vi "read_mote.vi"() -> (0 "DataSocket error":errorcluster, 1 "SF error":errorcluster, 3 "Timestamp":string)   [LabVIEW 2011]
panel:
  out "Location":string
  out "# Sent Data":u64
  out "Data comming from mote":string
  out "Deque error":errorcluster
  # "DO NOT USE id 0 for a mote !"
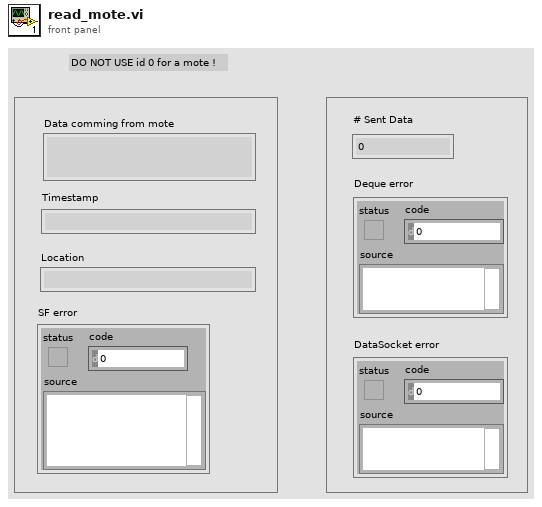
[diagram p1: front panel]
types:
  T1 = enum16{"Read", "Write", "ReadWrite", "BufferedRead", "BufferedReadWrite"}
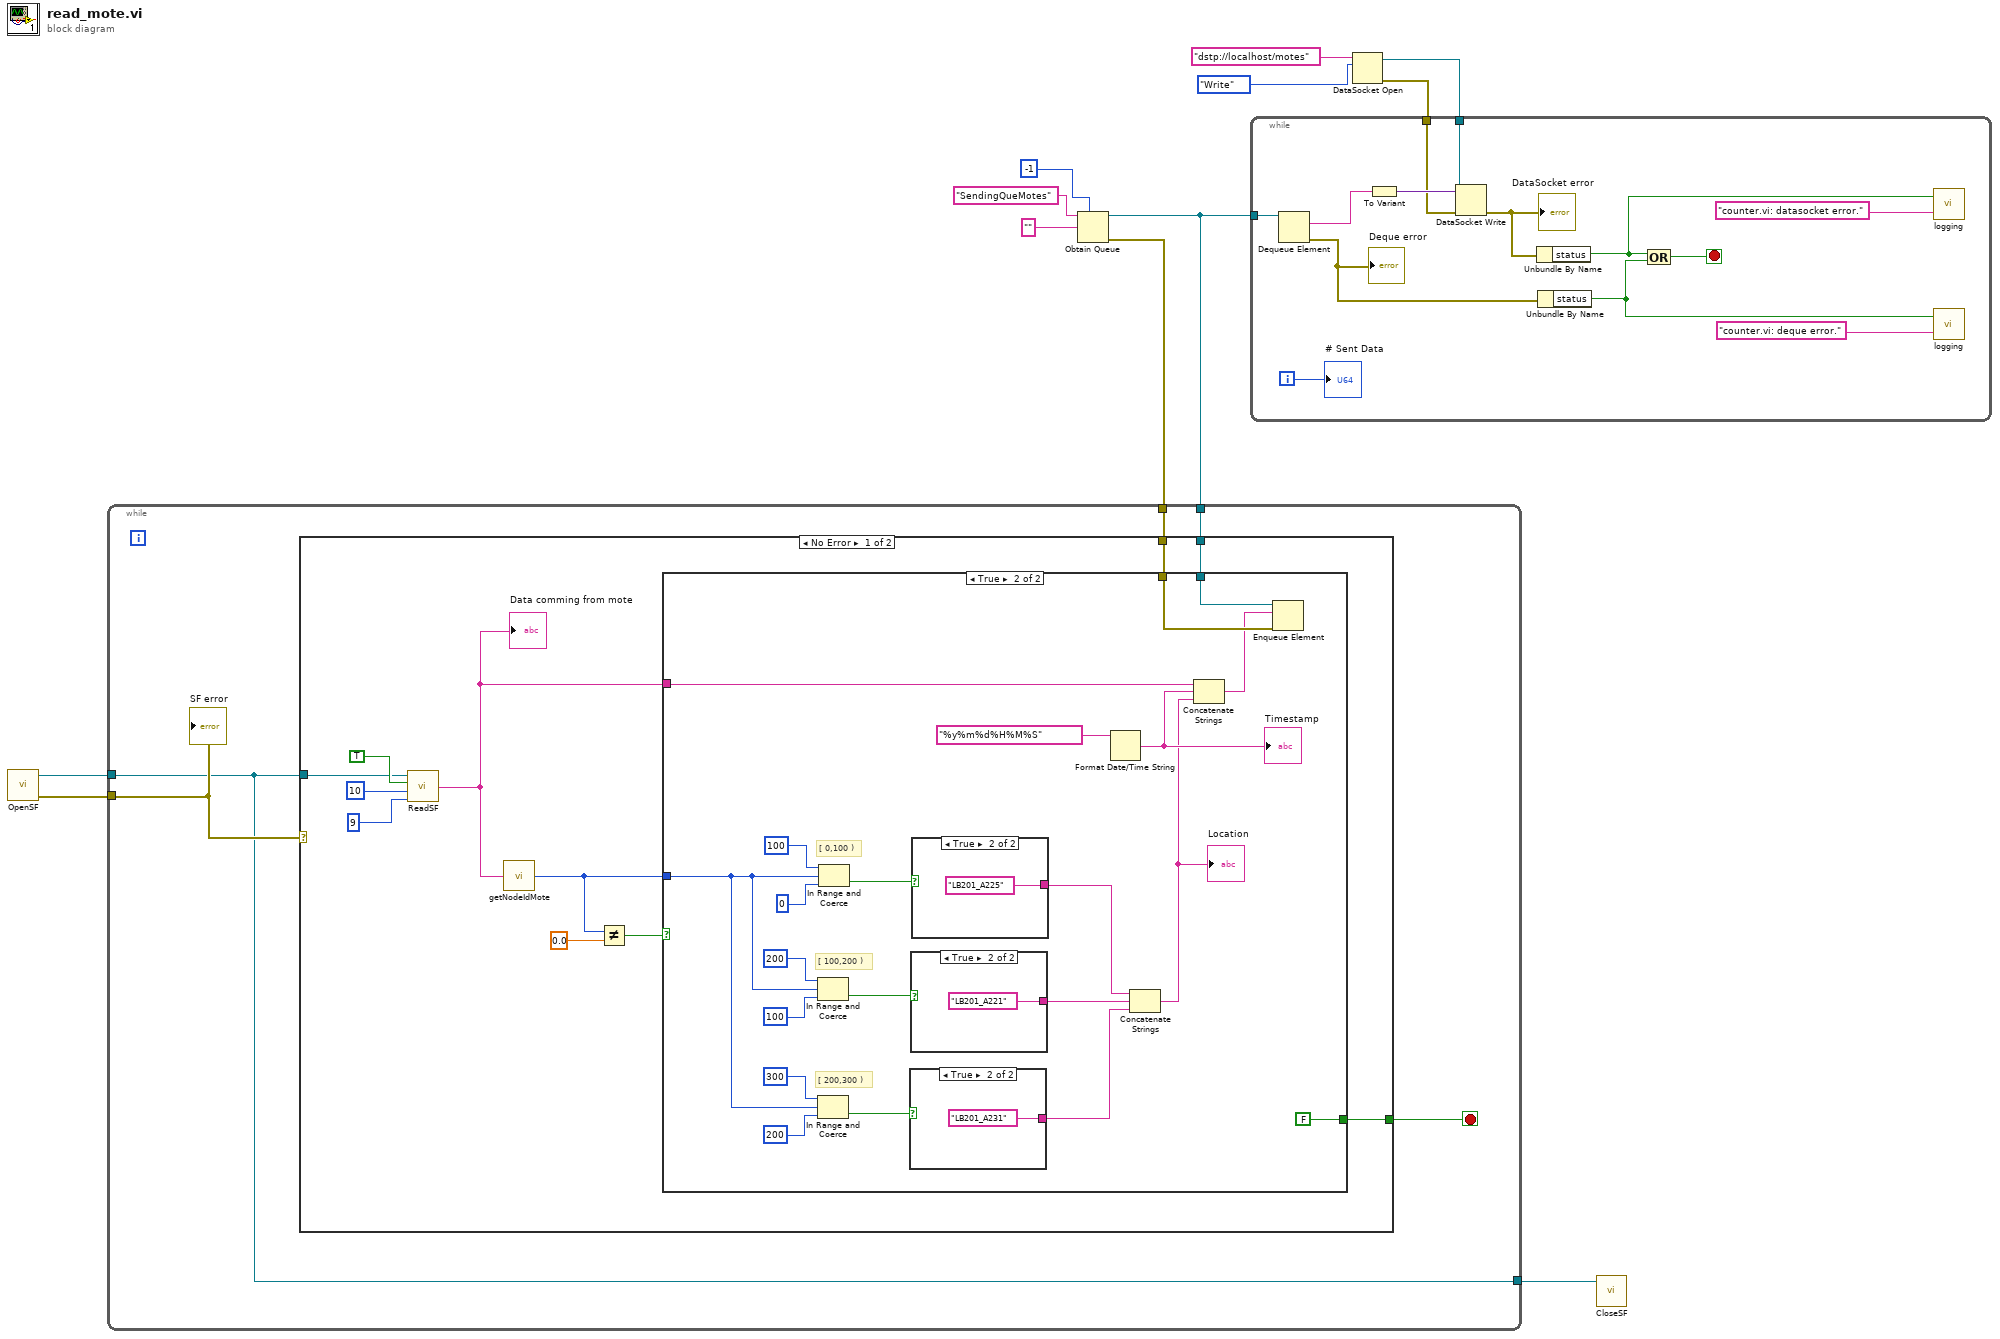
[diagram p0: block diagram]
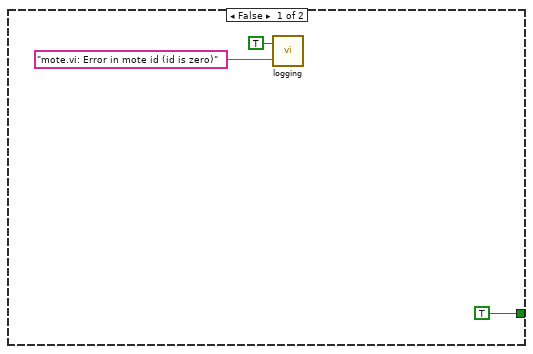
[diagram p2: hidden frame]
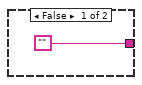
[diagram p3: hidden frame]
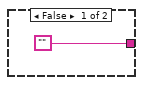
[diagram p4: hidden frame]
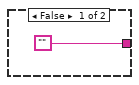
[diagram p5: hidden frame]
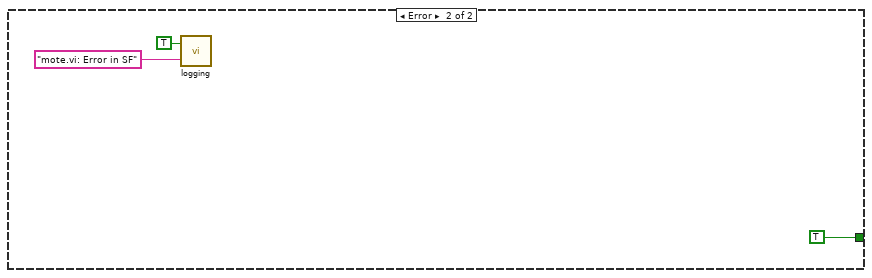
[diagram p6: hidden frame]
diagram:
  n1 = call "OpenSF.vi"() -> ("error out"=w3:errorcluster, "connection ID"=w2:refnum<k5>)  [unwired: 1 out]
  n2 = Obtain Queue(max queue size (-1, unlimited)=-1, name (unnamed)="SendingQueMotes", element data type="") -> (queue out=w5:refnum<queue>, error out=w6:errorcluster)  [unwired: 2 in, 1 out]
  n3 = while {
    tunnel: w2 -> [w14]
    tunnel: w3 -> [w15]
    tunnel: w6 -> [w17]
    tunnel: w5 -> [w16]
    tunnel: [w14] -> w1
    stop <- w13 stop-if-true
    n4 = case shown="No Error" w15 {
      tunnel: w14 -> [w25 _]
      tunnel: w17 -> [w24 _]
      tunnel: w16 -> [w23 _]
      tunnel: [w18 TRUE] -> w13
      frame No Error {
        n5 = call "ReadSF.vi"("connection ID in"=w25, "enabled"=TRUE, "bytes to read"=10 ("f"), "header size"=9 ("bytes to read")) -> ("string"=w22:string)  [unwired: 2 in, 2 out]
        "Data comming from mote" <- w22
        n6 = call "getNodeIdMote.vi"("input data"=w22) -> ("node id (1 byte)"=w21:u8)
        n7 = Not Equal?(x=w21, y=0.0 ("x")) -> (x != y?=w19:bool)
        n8 = case shown="True" w19 {
          tunnel: w24 -> [_ w51]
          tunnel: w23 -> [_ w50]
          tunnel: w22 -> [_ w47]
          tunnel: w21 -> [_ w33]
          tunnel: [TRUE FALSE] -> w18
          frame False {
            n9 = call "logging.vi"("data"="mote.vi: Error in mote id (id is zero)", "Boolean"=TRUE ("Enable")) -> ()  [unwired: 1 in]
          }
          frame True {
            # "[ 200,300 )"
            # "[ 100,200 )"
            # "[ 0,100 )"
            n10 = In Range and Coerce(upper limit=u64 200, x=w33, lower limit=u64 100) -> (In Range?=w39:bool)  [unwired: 1 out]
            n11 = In Range and Coerce(upper limit=u64 300, x=w33, lower limit=u64 200) -> (In Range?=w38:bool)  [unwired: 1 out]
            n12 = In Range and Coerce(upper limit=u64 100, x=w33, lower limit=u64 0) -> (In Range?=w40:bool)  [unwired: 1 out]
            n13 = case shown="True" w38 {
              tunnel: ["" "LB201_A231"] -> w35
              frame False {
              }
              frame True {
              }
            }
            n14 = case shown="True" w39 {
              tunnel: ["" "LB201_A221"] -> w36
              frame False {
              }
              frame True {
              }
            }
            n15 = case shown="True" w40 {
              tunnel: ["" "LB201_A225"] -> w37
              frame False {
              }
              frame True {
              }
            }
            n16 = Format Date/Time String(time format string (%c)="%y%m%d%H%M%S") -> (date/time string=w48:string)  [unwired: 2 in]
            "Timestamp" <- w48
            n17 = Concatenate Strings(w37, w36, w35) -> (w34:string)
            "Location" <- w34
            n18 = Concatenate Strings(w47, w48, w34) -> (w49:string)
            n19 = Enqueue Element(queue=w50, element=w49, error in (no error)=w51) -> ()  [unwired: 1 in, 3 out]
          }
        }
      }
      frame Error {
        n20 = call "logging.vi"("data"="mote.vi: Error in SF", "Boolean"=TRUE ("Enable")) -> ()  [unwired: 1 in]
      }
    }
    "SF error" <- w15
  }
  n21 = DataSocket Open(10:T1."Write" ("mode"), 11:"dstp://localhost/motes" ("URL 3")) -> (0:w7:errorcluster, 3:w8:refnum<k13>)  [unwired: 2 in]
  n22 = while {
    tunnel: w5 -> [w74]
    tunnel: w8 -> [w73]
    tunnel: w7 -> [w68]
    i -> [w67]
    stop <- w62 stop-if-true
    n23 = Dequeue Element(queue=w74) -> (element=w71:string, error out=w70:errorcluster)  [unwired: 2 in, 2 out]
    "Deque error" <- w70
    n24 = To Variant(anything=w71) -> (Variant=w72:variant)
    n25 = DataSocket Write(8:w68, 10:w72, 11:w73) -> (0:w69:errorcluster)  [unwired: 3 out]
    "DataSocket error" <- w69
    n26 = Unbundle By Name(w69) -> ("status"=w64:bool)
    n27 = Unbundle By Name(w70) -> ("status"=w63:bool)
    n28 = Compound Arithmetic op=OR(w64, w63) -> (w62:bool)
    n29 = call "logging.vi"("data"="counter.vi: datasocket error.", "Boolean"=w64) -> ()  [unwired: 1 in]
    n30 = call "logging.vi"("data"="counter.vi: deque error.", "Boolean"=w63) -> ()  [unwired: 1 in]
    "# Sent Data" <- w67
  }
  n31 = call "CloseSF.vi"("connection ID"=w1) -> ()  [unwired: 2 in]
